vi "Config VI.vi"(8 "error in (no error)":errorcluster, 11 "Plugin in":refnum<class "Plugin.lvclass">) -> (0 "error out":errorcluster, 3 "Plugin out":refnum<class "Plugin.lvclass">)   [LabVIEW 2015, in "JsonReportPlugin.lvclass"]
uses:
  JsonReportPlugin.lvclass
  Core/Plugin.lvclass
  Core/Plugin/Plugin Config UI State.ctl
panel:
  in  "Enable":bool
  in  "Include Result":bool
  in  "Include Timestamp":bool
  in  "Include SN":bool
  in  "Report Folder":string
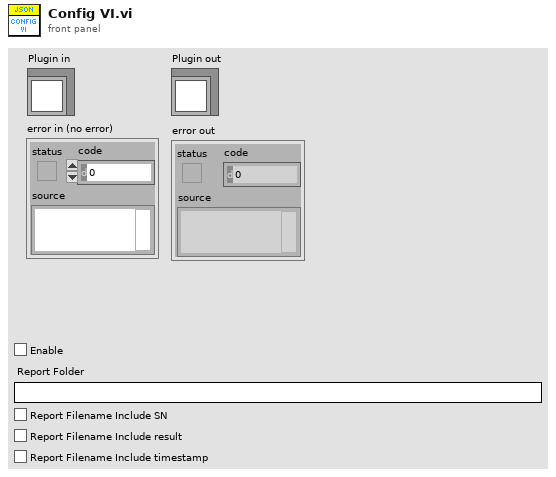
[diagram p1: front panel]
types:
  T1 = typedef "Plugin.lvclass/Plugin Config UI State.ctl" = enum16{"UI_LOOP", "INIT", "END"}
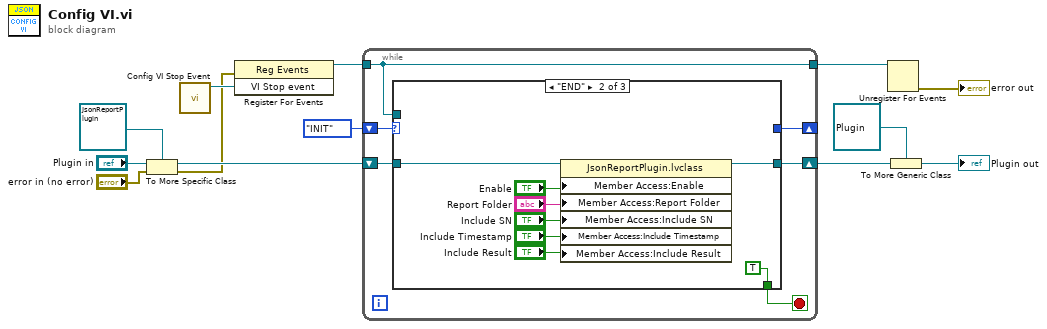
[diagram p0: block diagram]
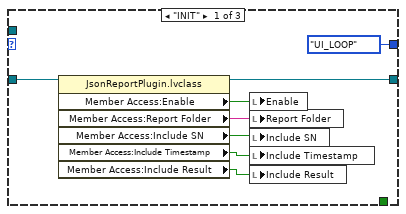
[diagram p2: hidden frame]
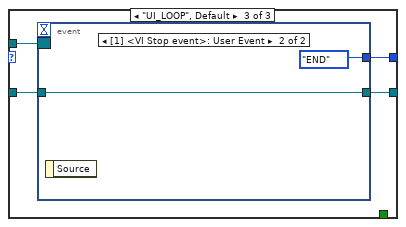
[diagram p3: hidden frame]
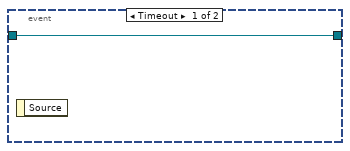
[diagram p4: hidden frame]
diagram:
  n1 = To More Specific Class(target class=refnum<class "JsonReportPlugin.lvclass"> refnum ("JsonReportPlugin.lvclass"), reference="Plugin in", error in="error in (no error)") -> (specific class reference=w9:refnum<class "JsonReportPlugin.lvclass">, error out=w3:errorcluster)
  n2 = call "Config VI Stop Event.vi"() -> ("VI Stop event"=w13:refnum<user-event>)  [unwired: 11 in]
  n3 = register-events(error in=w3, w13) -> (reference out=w12:refnum<event-registration>)  [unwired: 1 in, 1 out]
  n4 = while {
    tunnel: w12 -> [w18]
    tunnel: [w18] -> w6
    shift-right: [w16] -> _
    shift-left: Plugin_Config_UI_State."INIT" ("State") -> [w17]
    shift-right: [w14] -> w8
    shift-left: w9 -> [w15]
    stop <- w19 stop-if-true
    n5 = case shown="\"END\"" w17 {
      tunnel: [_ TRUE _] -> w19
      tunnel: w18 -> [_ _ w39]
      tunnel: [Plugin_Config_UI_State."UI_LOOP" ("State") _ w38] -> w16
      tunnel: w15 -> [w26 w34 w37]
      tunnel: [w25 w33 w36] -> w14
      frame "INIT" {
        n6 = property class="JsonReportPlugin.lvclass"(reference=w26) -> (reference out=w25:refnum<class "JsonReportPlugin.lvclass">, "Member Access:Enable"=w24:bool, "Member Access:Report Folder"=w23:string, "Member Access:Include SN"=w22:bool, "Member Access:Include Timestamp"=w21:bool, "Member Access:Include Result"=w20:bool)  [unwired: 1 in, 1 out]
        n7 = local write "Enable"(w24) -> ()
        n8 = local write "Report Folder"(w23) -> ()
        n9 = local write "Include SN"(w22) -> ()
        n10 = local write "Include Timestamp"(w21) -> ()
        n11 = local write "Include Result"(w20) -> ()
      }
      frame "END" {
        n12 = property class="JsonReportPlugin.lvclass"(reference=w34, "Member Access:Enable"="Enable", "Member Access:Report Folder"="Report Folder", "Member Access:Include SN"="Include SN", "Member Access:Include Timestamp"="Include Timestamp", "Member Access:Include Result"="Include Result") -> (reference out=w33:refnum<class "JsonReportPlugin.lvclass">)  [unwired: 1 in, 1 out]
      }
      frame "UI_LOOP", Default {
        n13 = event shown="[1] <VI Stop event>: User Event" {
          selector: w39 -> [_ _]
          dyn-events: _ -> [_ _]
          timeout: _ -> [_ _]
          tunnel: [_ Plugin_Config_UI_State."END" ("State")] -> w38
          tunnel: w37 -> [w40 w41]
          tunnel: [w40 w41] -> w36
          event Timeout {
            n14 = event-data() -> ()  [unwired: 1 in, 1 out]
          }
          event User Event {
            n15 = event-data() -> ()  [unwired: 1 in, 1 out]
          }
        }
      }
    }
  }
  n16 = Unregister For Events(event registration refnum=w6) -> (error out=→"error out":errorcluster)  [unwired: 1 in]
  n17 = To More Generic Class(target class=refnum<class "Plugin.lvclass"> refnum ("Plugin out"), reference=w8) -> (generic class reference=→"Plugin out":refnum<class "Plugin.lvclass">)
